vi "REV2mDistanceSensor Initialize.vi"(9 "Profile":T3, 10 "Port":T2) -> (3 "REV2mDistanceSensorDevRef Out":T4)   [LabVIEW 2019, in "DistanceSensorDriver.lvlib"]
uses:
  DistanceSensorDriver.lvlib
  Typedef/REV2mDistanceSensorDevRef.ctl
  Typedef/Ports.ctl
  Typedef/RangeProfile.ctl
  Typedef/VL53L0X_DeviceInfo_t.ctl
panel:
  out "DeviceInfo":T1
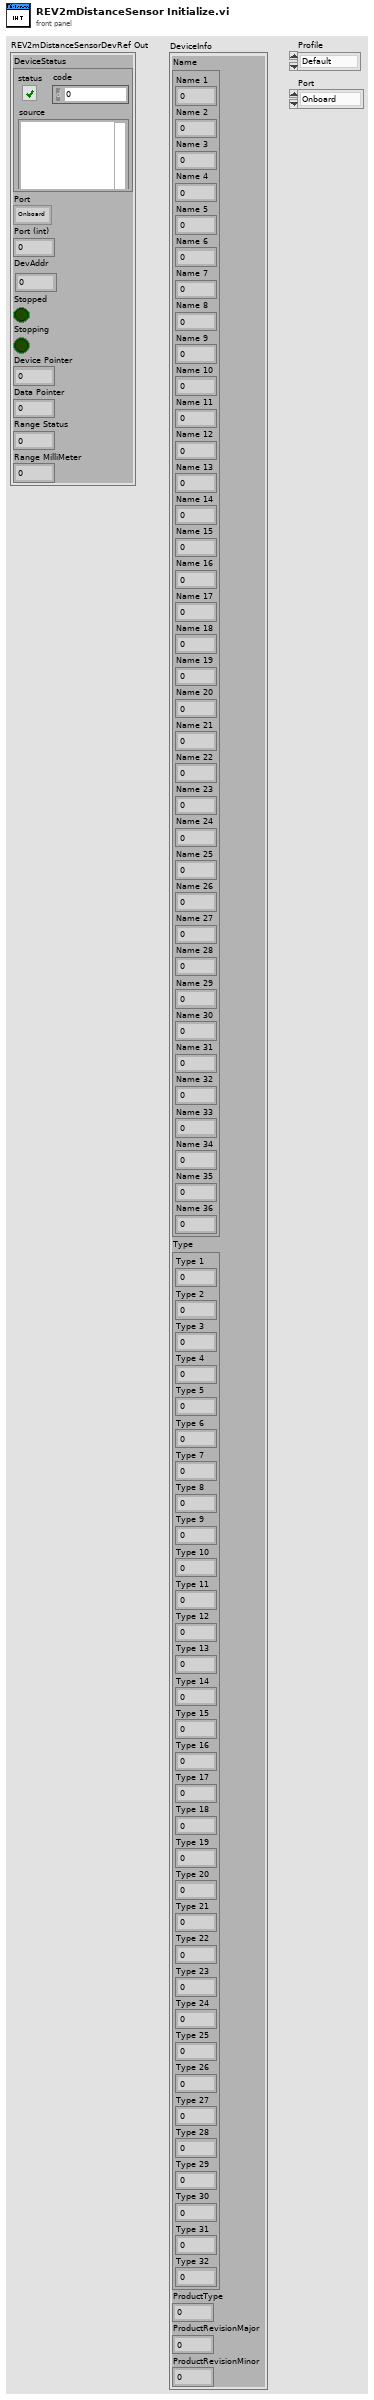
[diagram p1: front panel]
types:
  T1 = typedef "DistanceSensorDriver.lvlib/VL53L0X_DeviceInfo_t.ctl" = cluster{"Name":cluster{"Name 1":i8, "Name 2":i8, "Name 3":i8, "Name 4":i8, "Name 5":i8, "Name 6":i8, "Name 7":i8, "Name 8":i8, "Name 9":i8, "Name 10":i8, "Name 11":i8, "Name 12":i8, "Name 13":i8, "Name 14":i8, "Name 15":i8, "Name 16":i8, "Name 17":i8, "Name 18":i8, "Name 19":i8, "Name 20":i8, "Name 21":i8, "Name 22":i8, "Name 23":i8, "Name 24":i8, "Name 25":i8, "Name 26":i8, "Name 27":i8, "Name 28":i8, "Name 29":i8, "Name 30":i8, "Name 31":i8, "Name 32":i8, "Name 33":i8, "Name 34":i8, "Name 35":i8, "Name 36":i8}, "Type":cluster{"Type 1":i8, "Type 2":i8, "Type 3":i8, "Type 4":i8, "Type 5":i8, "Type 6":i8, "Type 7":i8, "Type 8":i8, "Type 9":i8, "Type 10":i8, "Type 11":i8, "Type 12":i8, "Type 13":i8, "Type 14":i8, "Type 15":i8, "Type 16":i8, "Type 17":i8, "Type 18":i8, "Type 19":i8, "Type 20":i8, "Type 21":i8, "Type 22":i8, "Type 23":i8, "Type 24":i8, "Type 25":i8, "Type 26":i8, "Type 27":i8, "Type 28":i8, "Type 29":i8, "Type 30":i8, "Type 31":i8, "Type 32":i8}, "ProductType":u8, "ProductRevisionMajor":u8, "ProductRevisionMinor":u8}
  T2 = typedef "DistanceSensorDriver.lvlib/Ports.ctl" = enum32{"Onboard", "MXP"}
  T3 = typedef "DistanceSensorDriver.lvlib/RangeProfile.ctl" = enum16{"Default", "High Speed", "High Accuracy", "Long Range"}
  T4 = typedef "DistanceSensorDriver.lvlib/REV2mDistanceSensorDevRef.ctl" = cluster{"DeviceStatus":errorcluster, "Port":T2, "Port (int)":i32, "DevAddr":i32, "Stopped":bool, "Stopping":bool, "Device Pointer":u64, "Data Pointer":u64, "Range Status":u8, "Range MilliMeter":u16}
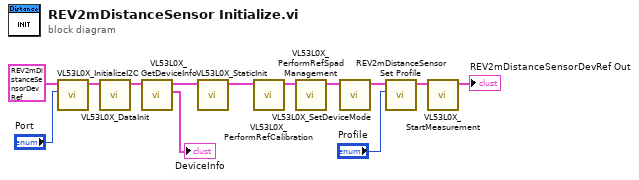
[diagram p0: block diagram]
diagram:
  n1 = call "VL53L0X_InitializeI2C.vi"("Port"="Port", "REV2mDistanceSensorDevRef"=T4 {"DeviceStatus"={"status"=FALSE, "code"=0, "source"=""}, "Port"=enum."Onboard", "Port (int)"=0, "DevAddr"=0, "Stopped"=FALSE, "Stopping"=FALSE, "Device Pointer"=0, "Data Pointer"=0, "Range Status"=0, "Range MilliMeter"=0}) -> ("REV2mDistanceSensorDevRef Out"=w8:T4)  [unwired: 9 in]
  n2 = call "VL53L0X_DataInit.vi"("REV2mDistanceSensorDevRef"=w8) -> ("REV2mDistanceSensorDevRef Out"=w5:T4)  [unwired: 10 in]
  n3 = call "VL53L0X_GetDeviceInfo.vi"("REV2mDistanceSensorDevRef"=w5) -> ("DeviceInfo"=→"DeviceInfo":T1, "REV2mDistanceSensorDevRef Out"=w3:T4)  [unwired: 9 in]
  n4 = call "VL53L0X_StaticInit.vi"("REV2mDistanceSensorDevRef"=w3) -> ("REV2mDistanceSensorDevRef Out"=w2:T4)  [unwired: 10 in]
  n5 = call "VL53L0X_PerformRefCalibration.vi"("REV2mDistanceSensorDevRef"=w2) -> ("REV2mDistanceSensorDevRef Out"=w7:T4)  [unwired: 8 in, 2 out]
  n6 = call "VL53L0X_PerformRefSpadManagement.vi"("REV2mDistanceSensorDevRef"=w7) -> ("REV2mDistanceSensorDevRef Out"=w6:T4)  [unwired: 8 in, 2 out]
  n7 = call "VL53L0X_SetDeviceMode.vi"("REV2mDistanceSensorDevRef"=w6) -> ("REV2mDistanceSensorDevRef Out"=w11:T4)  [unwired: 10 in]
  n8 = call "REV2mDistanceSensor Set Profile.vi"("Profile"="Profile", "REV2mDistanceSensorDevRef"=w11) -> ("REV2mDistanceSensorDevRef Out"=w12:T4)  [unwired: 9 in]
  n9 = call "VL53L0X_StartMeasurement.vi"("REV2mDistanceSensorDevRef"=w12) -> ("REV2mDistanceSensorDevRef Out"=→"REV2mDistanceSensorDevRef Out":T4)  [unwired: 10 in]
